vi "clase13_01_2021.vi"() -> ()   [LabVIEW 2020]
panel:
  in  "Numeric":i32
  out "Numeric 4":i32
  in  "Numeric 3":i32
  out "Numeric 2":dbl
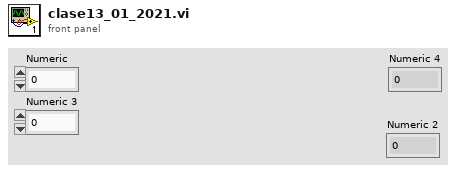
[diagram p1: front panel]
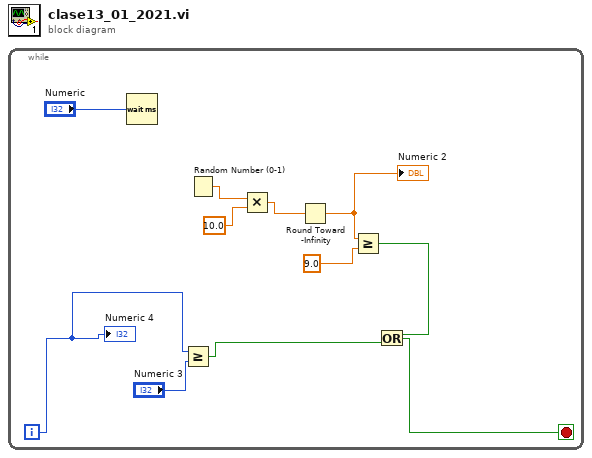
[diagram p0: block diagram]
diagram:
  n1 = while {
    i -> [w2]
    stop <- w4 stop-if-true
    n2 = Wait (ms)(milliseconds to wait="Numeric") -> ()  [unwired: 1 out]
    n3 = Greater Or Equal?(x=w2, y="Numeric 3") -> (x >= y?=w5:bool)
    n4 = Random Number (0-1)() -> (number: 0 to 1=w11:dbl)
    n5 = Multiply(x=w11, y=10.0) -> (x*y=w9:dbl)
    n6 = Round Toward -Infinity(1:w9) -> (0:w8:dbl)
    "Numeric 2" <- w8
    n7 = Greater Or Equal?(x=w8, y=9.0) -> (x >= y?=w6:bool)
    n8 = Or(x=w6, y=w5) -> (x .or. y?=w4:bool)
    "Numeric 4" <- w2
  }
